vi "Update Tag.vi"(7 "Index":i32, 8 "error in (no error)":errorcluster, 9 "Variant":variant, 10 "Tag ID / Name":variant, 11 "Raw Message in":refnum<class "Raw Message.lvclass">) -> (0 "error out":errorcluster, 2 "Key not found?":bool, 3 "Raw Message out":refnum<class "Raw Message.lvclass">)   [LabVIEW 2020, in "Protobuf RAW.lvlib" / "Raw Message.lvclass"]
uses:
  Raw Message.lvclass
  Raw Message.lvclass/Raw Message.ctl
  Tag/Basic Type.lvclass
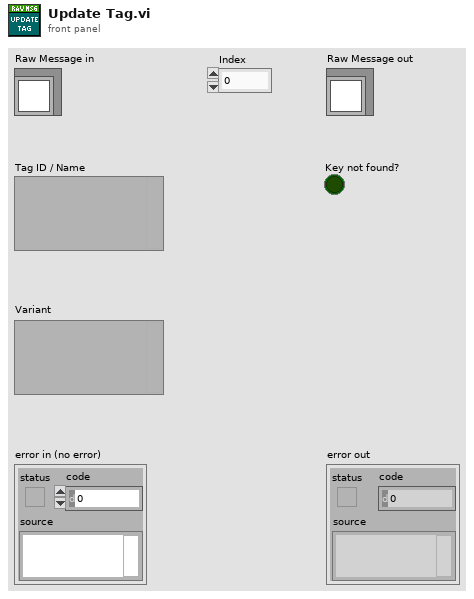
[diagram p1: front panel]
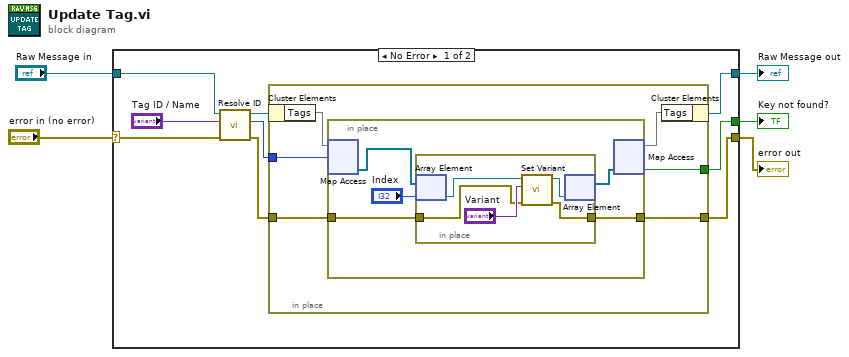
[diagram p0: block diagram]
diagram:
  n1 = case shown="No Error" "error in (no error)" {
    selector: "error in (no error)" -> [w13 w32]
    tunnel: [w12 w32] -> w4
    tunnel: [w14 w31] -> w2
    tunnel: "Raw Message in" -> [w9 w31]
    tunnel: [w11 _] -> w1
    frame No Error {
      n2 = call "Resolve ID.vi"("error in (no error)"=w13, "Tag ID / Name"="Tag ID / Name", "Raw Message in"=w9) -> ("error out"=w10:errorcluster, "Tag ID"=w6:u32, "Raw Message out"=w8:refnum<class "Raw Message.lvclass">)  [unwired: 6 in]
      n3 = in-place {
        in-place-border: w10 -> [w18]
        in-place-border: [w17] -> w12
        in-place-border: [w16] -> w11
        in-place-border: w6 -> [w15]
        n4 = in-place-cluster #1(w8) -> ("Tags"=w20:map{u32, refnum<class "Basic Type.lvclass">[]})
        n5 = in-place {
          in-place-border: w18 -> [w23]
          in-place-border: [w22] -> w17
          n6 = in-place-map #2(w20, w15) -> (w25:refnum<class "Basic Type.lvclass">[])  [unwired: 1 in, 1 out]
          n7 = in-place {
            in-place-border: w23 -> [w27]
            in-place-border: [w26] -> w22
            n8 = in-place-array #3(w25, "Index") -> (w30:refnum<class "Basic Type.lvclass">)
            n9 = call-dynamic "Set Variant.vi"("error in (no error)"=w27, "Variant"="Variant", "Type Serializer in"=w30) -> ("error out"=w26:errorcluster, "Type Serializer out"=w29:refnum<class "Basic Type.lvclass">)  [unwired: 7 in]
            n10 = in-place-array #3(w29) -> (w24:refnum<class "Basic Type.lvclass">[])  [unwired: 1 out]
          }
          n11 = in-place-map #2(w24) -> (w19:map{u32, refnum<class "Basic Type.lvclass">[]}, w16:bool)  [unwired: 1 in, 1 out]
        }
        n12 = in-place-cluster #1("Tags"=w19) -> (w14:refnum<class "Raw Message.lvclass">)
      }
    }
    frame Error {
    }
  }
  "error out" <- w4
  "Raw Message out" <- w2
  "Key not found?" <- w1
